vi "MCD (FPGA).vi"() -> ()   [LabVIEW 2012]
doc: "This VI uses 2 derived clocks as timing sources to 2 independent single-cycle timed loops. The VI also has a normal while loop that runs at the top-level clock rate."
uses:
  <vilib>/Platform/TimedLoop/XDataNode/timing_clust.ctl
  <vilib>/Platform/TimedLoop/XDataNode/nitl_modes.ctl
  <vilib>/Platform/TimedLoop/XDataNode/wakeup.ctl
  <vilib>/rvi/Emulation/niFpgaSctlEmulationRegisterWithScheduler.vi
  <vilib>/rvi/Emulation/niFpgaSctlEmulationScheduler.vi
  <vilib>/Platform/TimedLoop/XDataNode/XDataNode.xnode
  <vilib>/Platform/TimedLoop/XDataNode/XDNodeRunTimeDep.lvlib
panel:
  out "SCTL 120MHz":u32
  out "SCTL 13.33MHz":u32
  out "Normal Loop 40MHz":u32
  in  "stop":bool
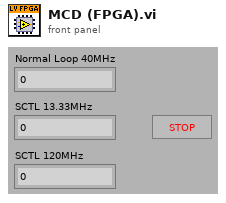
[diagram p1: front panel]
types:
  T1 = typedef "XDNodeRunTimeDep.lvlib/timing_clust.ctl" = cluster{"Expected End [f-1]":u64, "Actual End [f-1]":u64, "Finished Late? [f-1]":bool, "Expected End [i-1]":u64, "Actual End [i-1]":u64, "Finished Late? [i-1]":bool, "Expected Start [i]":u64, "Actual Start [i]":u64, "Expected Start [f]":u64, "Actual Start [f]":u64, "Source Name":string, "Structure Name":string, "Period":i64, "Deadline":i64, "Offset":i64, "Start":i64, "Priority":i32, "Timeout":i32, "Mode":T2, "Wakeup Reason":T3, "Error":errorcluster, "Source Type":string, "Secondary Source Type":string, "Global End Time":u64, "Global Start Time":u64, "Frame Duration":u64, "Iteration Duration":u64, "Assigned CPU":i32, "I/O Scan Engine Mode":u32}
  T2 = typedef "XDNodeRunTimeDep.lvlib/nitl_modes.ctl" = enum32{"No Change", "Process missed periods, maintain original phase", "Discard missed periods, maintain original phase", "Process missed periods, ignore original phase", "Discard missed periods, ignore original phase"}
  T3 = typedef "XDNodeRunTimeDep.lvlib/wakeup.ctl" = enum32{"Normal", "Aborted", "Asynchronous wakeup", "Timing source error", "Timed loop error", "Timeout"}
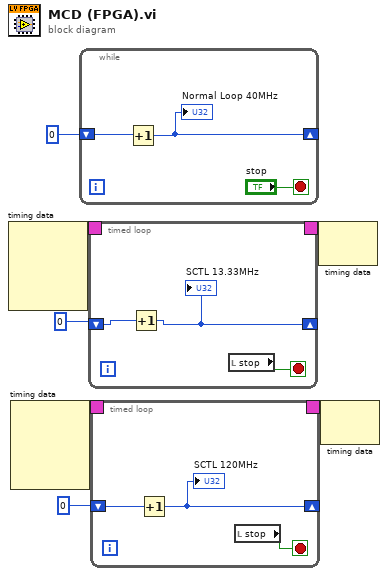
[diagram p0: block diagram]
diagram:
  n1 = node-c288() -> (w7:T1)  [unwired: 4 out]
  n2 = node-c288() -> (w5:T1)  [unwired: 4 out]
  n3 = while {
    shift-right: [w9] -> _
    shift-left: u32 0 -> [w10]
    stop <- "stop" stop-if-true
    n4 = Increment(x=w10) -> (x+1=w9:u32)
    "Normal Loop 40MHz" <- w9
  }
  n5 = timed-loop {
    timing: w7 -> [_]
    timing-out: [_] -> w6
    shift-right: [w12] -> _
    shift-left: u32 0 -> [w13]
    stop <- w11 stop-if-true
    n6 = Increment(x=w13) -> (x+1=w12:u32)
    "SCTL 13.33MHz" <- w12
    n7 = local read "stop"() -> (w11:bool)
  }
  n8 = timed-loop {
    timing: w5 -> [_]
    timing-out: [_] -> w4
    shift-right: [w17] -> _
    shift-left: u32 0 -> [w18]
    stop <- w16 stop-if-true
    n9 = Increment(x=w18) -> (x+1=w17:u32)
    "SCTL 120MHz" <- w17
    n10 = local read "stop"() -> (w16:bool)
  }
  n11 = node-c288(w6) -> ()  [unwired: 1 out]
  n12 = node-c288(w4) -> ()  [unwired: 1 out]
